vi "STM Write Msg.vi"(7 "Meta data":T1[](array[typedef]), 8 "error in (no error)":errorcluster, 9 "Data":string, 10 "Name":string, 11 "connection ID":refnum<k5>) -> (0 "error out":errorcluster, 3 "connection ID out":refnum<k5>)   [LabVIEW 2014, in "QwaveSys Raspberry Pi Library.lvlib"]
doc: "This VI writes a package of data to a remote computer. It prepends a meta data ID number to each packet. \n\nThe data must be passed in as a String. The calling VI is responsible for flattening the desired data to a string before passing it to this VI."
uses:
  _SubVIs/TypeDefs/stm_MetaElement.ctl
  QwaveSys Raspberry Pi Library.lvlib
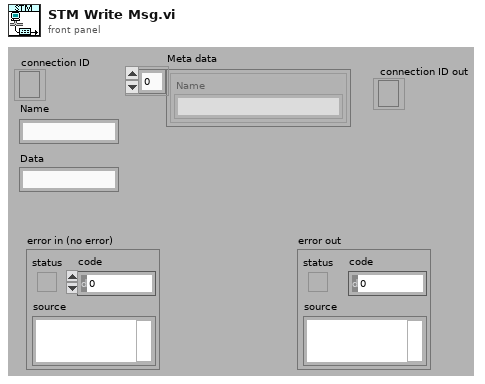
[diagram p1: front panel]
types:
  T1 = typedef "QwaveSys Raspberry Pi Library.lvlib/stm_MetaElement.ctl" = cluster{"Name":string}
  T2 = typedef "QwaveSys Raspberry Pi Library.lvlib/stm_MetaID.ctl" = u16
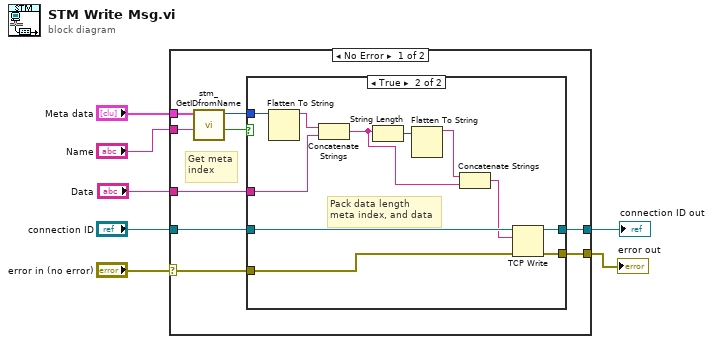
[diagram p0: block diagram]
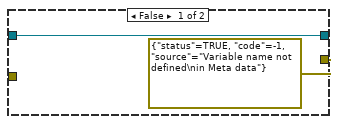
[diagram p2: hidden frame]
diagram:
  n1 = case shown="No Error" "error in (no error)" {
    selector: "error in (no error)" -> [w8 w31]
    tunnel: "connection ID" -> [w16 w30]
    tunnel: [w15 w31] -> w6
    tunnel: [w14 w30] -> w5
    tunnel: "Meta data" -> [w13 _]
    tunnel: "Name" -> [w12 _]
    tunnel: "Data" -> [w10 _]
    frame No Error {
      # "Get meta\nindex"
      n2 = call "stm_GetIDfromName.vi"("Name"=w12, "MetaData"=w13) -> ("Found"=w9:bool, "Meta ID"=w11:T2)  [unwired: 8 out]
      n3 = case shown="True" w9 {
        tunnel: w16 -> [w18 w29]
        tunnel: w8 -> [_ w28]
        tunnel: [errorcluster {"status"=TRUE, "code"=-1, "source"="Variable name not defined\nin Meta data"} ("error out") w27] -> w15
        tunnel: [w18 w26] -> w14
        tunnel: w11 -> [_ w25]
        tunnel: w10 -> [_ w21]
        frame False {
        }
        frame True {
          # "Pack data length\nmeta index, and data"
          n4 = Flatten To String(anything=w25) -> (data string=w24:string)  [unwired: 1 in, 4 out]
          n5 = Concatenate Strings(w24, w21) -> (w22:string)
          n6 = String Length(string=w22) -> (length=w23:i32)
          n7 = Flatten To String(anything=w23) -> (data string=w20:string)  [unwired: 1 in, 4 out]
          n8 = Concatenate Strings(w20, w22) -> (w19:string)
          n9 = TCP Write(connection ID=w29, data in=w19, error in (no error)=w28) -> (connection ID out=w26:refnum<k5>, error out=w27:errorcluster)  [unwired: 2 out]
        }
      }
    }
    frame Error {
    }
  }
  "error out" <- w6
  "connection ID out" <- w5
